vi "Set Waveform Type [AWF].vi"(7 "Micropulse # In":i32, 8 "error in (no error)":errorcluster, 9 "Waveform Type":T1, 11 "Test Number":u32) -> (0 "error out":errorcluster, 5 "Micropulse # Out":i32)   [LabVIEW 2026, in "MicroPulse_Driver.lvlib"]
doc: "Selects for test specified the analogue input signal for the signal processing.\n\nParameters:\n<Tn> : Test number. An integer value from 0 to the maximum number of tests (default maximum is 1279 tests).\nTn = 0 for all conventional tests. If the S extension is used it applies to all tests in the sweep number specified: 1-32, 0 = all sweeps.\n\n<Value> : \n0 – display and process rectified signal.\n1 – display and process full RF signal.\n2 – +ve half wave.\n3 – -ve half wave.\n\nExamples:\nAWF 5 0 : Set Test 5 to display and process rectified Ultrasonic signal.\nAWF 3 1 : Set Test 3 to display and process Full Wave RF Ultrasonic signal.\nAWF 0 0 : Set all tests to display and process rectified Ultrasonic signal."
uses:
  MicroPulse_Driver.lvlib
  <instrlib>/MicroPulse/Public/Data/Datatypes/MP - waveform type.ctl
  Private/MP-Registry Action-Enum.ctl
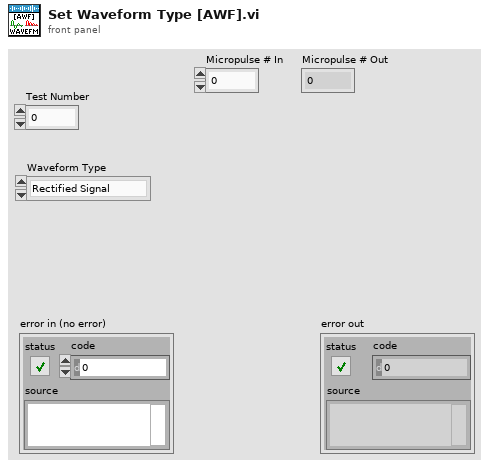
[diagram p1: front panel]
types:
  T1 = typedef "MicroPulse_Driver.lvlib/MP - waveform type.ctl" = enum16{"Rectified Signal", "RF Signal", "+Half Wave", "-Half Wave"}
  T2 = typedef "MicroPulse_Driver.lvlib/MP-Registry Action-Enum.ctl" = enum16{"Read", "Add Test", "Add Command", "Add Gate Command", "Add Encoder Command", "Clear Command  List", "Set Registry", "Set System Details", "Set DOF", "Set Velocity", "Disable Asynch Reads", "Enable Asynch Reads", "Add Connection", "Disconnect", "Shutdown"}
  T3 = typedef "MicroPulse_Driver.lvlib/TCP config.ctl" = cluster{"Connection ID":refnum<k5>, "IP address":string, "host port":u16, "OC timeout":i32, "Read timeout":i32, "Write timeout":i32}
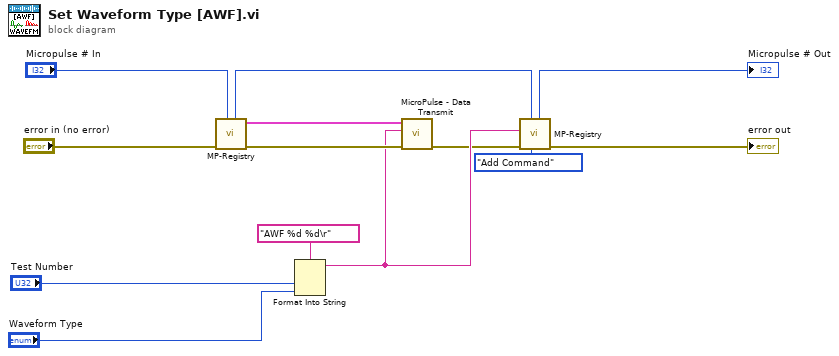
[diagram p0: block diagram]
diagram:
  n1 = call "MP-Registry.vi"("Micropulse # In"="Micropulse # In", "error in (no error)"="error in (no error)") -> ("error out"=w11:errorcluster, "TCP config"=w10:T3, "Micropulse # Out"=w4:i32)  [unwired: 6 in, 1 out]
  n2 = Format Into String(format string="AWF %d %d\r", "Test Number", "Waveform Type") -> (resulting string=w8:string)  [unwired: 2 in, 1 out]
  n3 = call "MicroPulse - Data Transmit.vi"("error in (no error)"=w11, "data"=w8, "TCP config"=w10) -> ("error out"=w6:errorcluster)  [unwired: 6 in, 2 out]
  n4 = call "MP-Registry.vi"("Action"=MP-Registry_Action-Enum."Add Command", "Micropulse # In"=w4, "error in (no error)"=w6, "Data in"=w8) -> ("error out"=→"error out":errorcluster, "Micropulse # Out"=→"Micropulse # Out":i32)  [unwired: 4 in, 2 out]
